vi "Update_Cuenta.vi"(8 "error in (no error)":errorcluster, 10 "Cuenta":bool[](array[boolean]), 11 "Contador_Bin_Actor in":refnum<class "Contador_Bin_Actor.lvclass">) -> (0 "error out":errorcluster, 3 "Contador_Bin_Actor out":refnum<class "Contador_Bin_Actor.lvclass">)   [LabVIEW 2019, in "Contador_Bin_Actor.lvlib" / "Contador_Bin_Actor.lvclass"]
uses:
  Contador_Bin_Actor.lvclass
  Contador_Bin_Actor.lvclass/Contador_Bin_Actor.ctl
  Logging_Contador_Actor/Logging_Contador_Actor Messages/Save_cuenta Msg/Save_cuenta Msg.lvclass/Save_cuenta Msg.ctl
  <vilib>/ActorFramework/Message Enqueuer/Message Enqueuer.lvclass/Message Enqueuer.ctl
  <vilib>/ActorFramework/Message Enqueuer/Enqueue.vi
  Logging_Contador_Actor/Logging_Contador_Actor Messages/Save_cuenta Msg/Save_cuenta Msg.lvclass
  C:/Program Files/National Instruments/LabVIEW 2019/vi.lib/ActorFramework/Message/Message.lvclass
  <vilib>/ActorFramework/Message Priority Queue/Priority Enqueue.vi
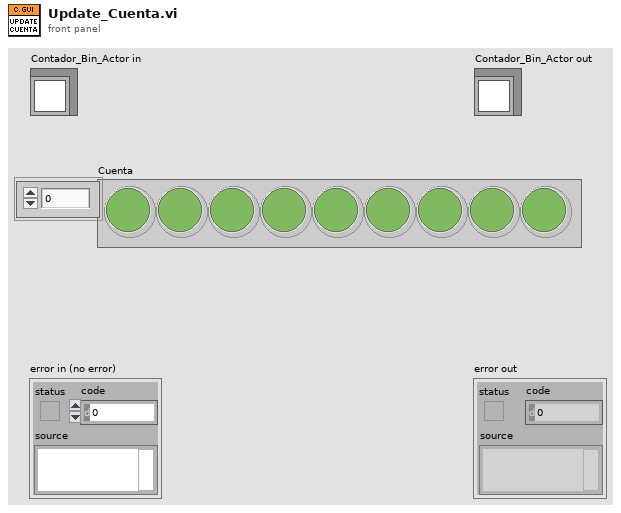
[diagram p1: front panel]
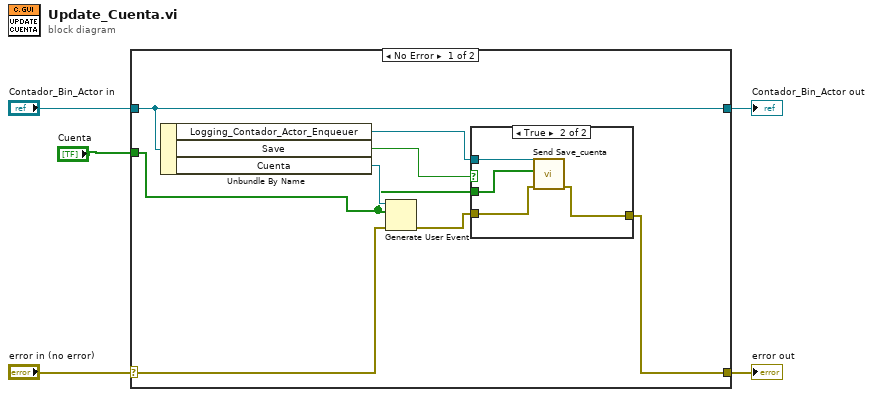
[diagram p0: block diagram]
diagram:
  n1 = case shown="No Error" "error in (no error)" {
    selector: "error in (no error)" -> [w11 w20]
    tunnel: [w6 w20] -> w4
    tunnel: [w13 w19] -> w2
    tunnel: "Contador_Bin_Actor in" -> [w13 w19]
    tunnel: "Cuenta" -> [w8 _]
    frame No Error {
      n2 = Unbundle By Name(w13) -> ("Logging_Contador_Actor_Enqueuer"=w9:refnum<class "Message Enqueuer.lvclass">, "Save"=w10:bool, "Cuenta"=w12:refnum<user-event>)
      n3 = Generate User Event(user event=w12, event data cluster=w8, error in=w11) -> (error out=w7:errorcluster)  [unwired: 1 in, 1 out]
      n4 = case shown="True" w10 {
        tunnel: w9 -> [_ w18]
        tunnel: w8 -> [_ w17]
        tunnel: w7 -> [w14 w16]
        tunnel: [w14 w15] -> w6
        frame False {
        }
        frame True {
          n5 = call "Send Save_cuenta.vi"("error in (no error)"=w16, "Cuenta"=w17, "Message Enqueuer"=w18) -> ("error out"=w15:errorcluster)  [unwired: 7 in, 1 out]
        }
      }
    }
    frame Error {
    }
  }
  "error out" <- w4
  "Contador_Bin_Actor out" <- w2
